vi "Evaluate.vi"(8 "error in (no error)":errorcluster, 10 "Variable Values":dbl[](array[numeric]), 11 "Expression":T1) -> (0 "error out":errorcluster, 3 "Evaluated":dbl)   [LabVIEW 2022 SP3, in "Expressions.lvlib"]
uses:
  Expressions.lvlib
  Controls/Expression.ctl
  Controls/Token Type.ctl
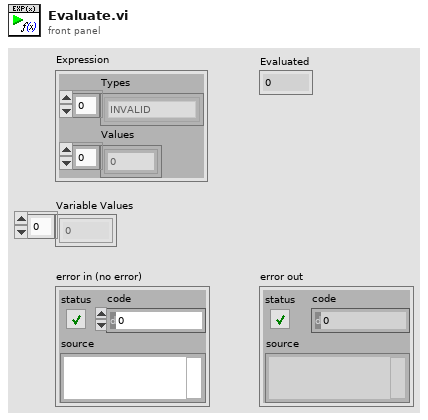
[diagram p1: front panel]
types:
  T1 = typedef "Expressions.lvlib/Expression.ctl" = cluster{"Types":T2[], "Values":dbl[]}
  T2 = typedef "Expressions.lvlib/Token Type.ctl" = enum8{"INVALID", "NOT", "AND", "OR", "EE", "NE", "LT", "GT", "LTE", "GTE", "PLUS", "MINUS", "MULTIPLY", "DIVIDE", "MODULUS", "LPAREN", "RPAREN", "LITERAL", "IDENTIFIER", "DEFINITION"}
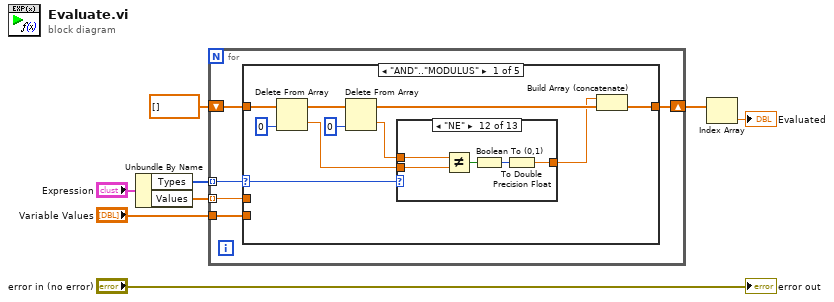
[diagram p0: block diagram]
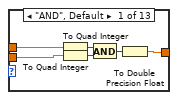
[diagram p2: hidden frame]
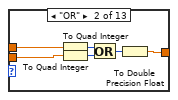
[diagram p3: hidden frame]
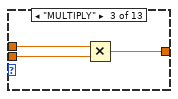
[diagram p4: hidden frame]
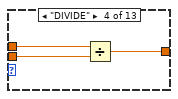
[diagram p5: hidden frame]
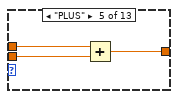
[diagram p6: hidden frame]
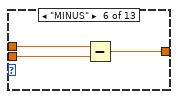
[diagram p7: hidden frame]
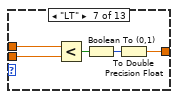
[diagram p8: hidden frame]
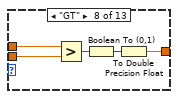
[diagram p9: hidden frame]
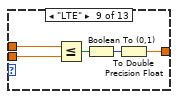
[diagram p10: hidden frame]
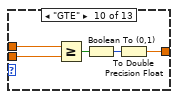
[diagram p11: hidden frame]
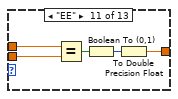
[diagram p12: hidden frame]
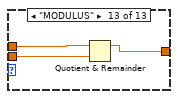
[diagram p13: hidden frame]
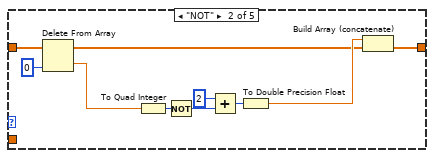
[diagram p14: hidden frame]
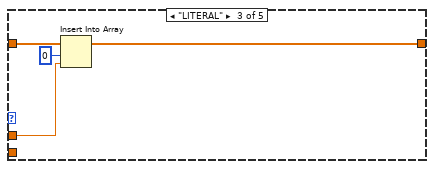
[diagram p15: hidden frame]
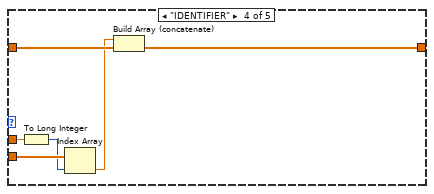
[diagram p16: hidden frame]
diagram:
  n1 = Unbundle By Name("Expression") -> ("Types"=w4:T2[], "Values"=w3:dbl[])
  n2 = for {
    shift-right: [w13] -> w2
    shift-left: dbl[] [] -> [w12]
    tunnel: "Variable Values" -> [w11]
    tunnel: w4 -> [w10] mode=indexing
    tunnel: w3 -> [w9] mode=indexing
    n3 = case shown="\"AND\"..\"MODULUS\"" w10 {
      selector: w10 -> [w14 _ _ _ _]
      tunnel: w9 -> [_ _ w91 w96 _]
      tunnel: [w19 w88 w94 w97 w101] -> w13
      tunnel: w12 -> [w23 w90 w93 w99 w101]
      tunnel: w11 -> [_ _ _ w100 _]
      frame "AND".."MODULUS" {
        n4 = Delete From Array(array=w23, index=0) -> (deleted portion=w18:dbl, array with subset deleted=w21:dbl[])  [unwired: 1 in]
        n5 = Delete From Array(array=w21, index=0) -> (deleted portion=w15:dbl, array with subset deleted=w20:dbl[])  [unwired: 1 in]
        n6 = case shown="\"NE\"" w14 {
          tunnel: w18 -> [w29 w35 w37 w40 w43 w46 w51 w56 w61 w66 w71 w76 w79]
          tunnel: [w28 w34 w36 w39 w42 w45 w48 w53 w58 w63 w68 w73 w78] -> w17
          tunnel: w15 -> [w27 w33 w38 w41 w44 w47 w52 w57 w62 w67 w72 w77 w80]
          frame "AND", Default {
            n7 = To Quad Integer(1:w27) -> (0:w25:i64)
            n8 = To Quad Integer(1:w29) -> (0:w26:i64)
            n9 = And(x=w25, y=w26) -> (x .and. y?=w24:i64)
            n10 = To Double Precision Float(number=w24) -> (double precision float=w28:dbl)
          }
          frame "OR" {
            n11 = To Quad Integer(1:w33) -> (0:w31:i64)
            n12 = To Quad Integer(1:w35) -> (0:w32:i64)
            n13 = Or(x=w31, y=w32) -> (x .or. y?=w30:i64)
            n14 = To Double Precision Float(number=w30) -> (double precision float=w34:dbl)
          }
          frame "MULTIPLY" {
            n15 = Multiply(x=w38, y=w37) -> (x*y=w36:dbl)
          }
          frame "DIVIDE" {
            n16 = Divide(x=w41, y=w40) -> (x/y=w39:dbl)
          }
          frame "PLUS" {
            n17 = Add(x=w44, y=w43) -> (x+y=w42:dbl)
          }
          frame "MINUS" {
            n18 = Subtract(x=w47, y=w46) -> (x-y=w45:dbl)
          }
          frame "LT" {
            n19 = Less?(x=w52, y=w51) -> (x < y?=w50:bool)
            n20 = Boolean To (0,1)(Boolean=w50) -> (0, 1=w49:i16)
            n21 = To Double Precision Float(number=w49) -> (double precision float=w48:dbl)
          }
          frame "GT" {
            n22 = Greater?(x=w57, y=w56) -> (0:w55:bool)
            n23 = Boolean To (0,1)(Boolean=w55) -> (0, 1=w54:i16)
            n24 = To Double Precision Float(number=w54) -> (double precision float=w53:dbl)
          }
          frame "LTE" {
            n25 = Less Or Equal?(x=w62, y=w61) -> (x <= y?=w60:bool)
            n26 = Boolean To (0,1)(Boolean=w60) -> (0, 1=w59:i16)
            n27 = To Double Precision Float(number=w59) -> (double precision float=w58:dbl)
          }
          frame "GTE" {
            n28 = Greater Or Equal?(x=w67, y=w66) -> (x >= y?=w65:bool)
            n29 = Boolean To (0,1)(Boolean=w65) -> (0, 1=w64:i16)
            n30 = To Double Precision Float(number=w64) -> (double precision float=w63:dbl)
          }
          frame "EE" {
            n31 = Equal?(x=w72, y=w71) -> (x = y?=w70:bool)
            n32 = Boolean To (0,1)(Boolean=w70) -> (0, 1=w69:i16)
            n33 = To Double Precision Float(number=w69) -> (double precision float=w68:dbl)
          }
          frame "NE" {
            n34 = Not Equal?(x=w77, y=w76) -> (x != y?=w75:bool)
            n35 = Boolean To (0,1)(Boolean=w75) -> (0, 1=w74:i16)
            n36 = To Double Precision Float(number=w74) -> (double precision float=w73:dbl)
          }
          frame "MODULUS" {
            n37 = Quotient & Remainder(x=w80, y=w79) -> (x-y*floor(x/y)=w78:dbl)  [unwired: 1 out]
          }
        }
        n38 = Build Array (concatenate)(w17, w20) -> (w19:dbl[])
      }
      frame "NOT" {
        n39 = Delete From Array(array=w90, index=0) -> (deleted portion=w87:dbl, array with subset deleted=w85:dbl[])  [unwired: 1 in]
        n40 = To Quad Integer(1:w87) -> (0:w84:i64)
        n41 = Not(x=w84) -> (.not. x?=w83:i64)
        n42 = Add(x=i64 2, y=w83) -> (x+y=w81:i64)
        n43 = To Double Precision Float(number=w81) -> (double precision float=w86:dbl)
        n44 = Build Array (concatenate)(w86, w85) -> (w88:dbl[])
      }
      frame "LITERAL" {
        n45 = Insert Into Array(array=w93, index=0, new element=w91) -> (w94:dbl[])
      }
      frame "IDENTIFIER" {
        n46 = To Long Integer(number=w96) -> (32bit integer=w95:i32)
        n47 = Index Array(array=w100, index=w95) -> (element=w98:dbl)
        n48 = Build Array (concatenate)(w98, w99) -> (w97:dbl[])
      }
      frame "INVALID", "LPAREN", "RPAREN", "DEFINITION" {
      }
    }
  }
  n49 = Index Array(array=w2) -> (element=→"Evaluated":dbl)  [unwired: 1 in]
  "error out" <- "error in (no error)"
